vi "home arm.vi"(11 "Home":bool) -> ()   [LabVIEW 2017]
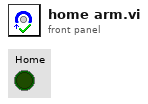
[diagram p1: front panel]
types:
  T1 = typedef "WPI_DigitalInputDevRef.ctl" = cluster{"DevStatus":errorcluster, "DIO Channel":T2}
  T2 = typedef "FPGA_DIOChannel.ctl" = enum8{"DIO 0", "DIO 1", "DIO 2", "DIO 3", "DIO 4", "DIO 5", "DIO 6", "DIO 7", "DIO 8", "DIO 9", "DIO MXP 0", "DIO MXP 1", "DIO MXP 2", "DIO MXP 3", "DIO MXP 4", "DIO MXP 5", "DIO MXP 6", "DIO MXP 7", "DIO MXP 8", "DIO MXP 9", "DIO MXP 10", "DIO MXP 11", "DIO MXP 12", "DIO MXP 13", "DIO MXP 14", "DIO MXP 15", "SPI Port CS1", "SPI Port CS2", "SPI Port CS3", "SPI Port MISO", "SPI Port MOSI", "Invalid"}
  T3 = typedef "WPI_MotorControlDeviceRef.ctl" = cluster{"DeviceStatus":errorcluster, "Type":T4, "PWM":cluster{"PWM Channel":T5, "DeadBand":T6}, "CAN":cluster{"Device Number":u8, "SetOutput VI Ref":variant, "GetOutput VI Ref":variant, "Enable VI Ref":variant, "Disable VI Ref":variant, "Data":variant}, "Invert":bool, "DIO PWM":cluster{"PWM \"Enable\" Channel":T5, "DIOChannel":T2, "PWM Rate":dbl}}
  T4 = typedef "WPI_MotorControlType.ctl" = enum16{"PWM", "CAN", "DIO PWM"}
  T5 = typedef "FPGA_DIOPWMChannel.ctl" = enum8{"PWM 0", "PWM 1", "PWM 2", "PWM 3", "PWM 4", "PWM 5", "PWM 6", "PWM 7", "PWM 8", "PWM 9", "PWM MXP 0", "PWM MXP 1", "PWM MXP 2", "PWM MXP 3", "PWM MXP 4", "PWM MXP 5", "PWM MXP 6", "PWM MXP 7", "PWM MXP 8", "PWM MXP 9", "Invalid"}
  T6 = typedef "WPI_PWMDeadband.ctl" = cluster{"Name":string, "maxPositivePwm":i32, "minPositivePwm":i32, "centerPwm":i32, "maxNegativePwm":i32, "minNegativePwm":i32, "angularRange":u16}
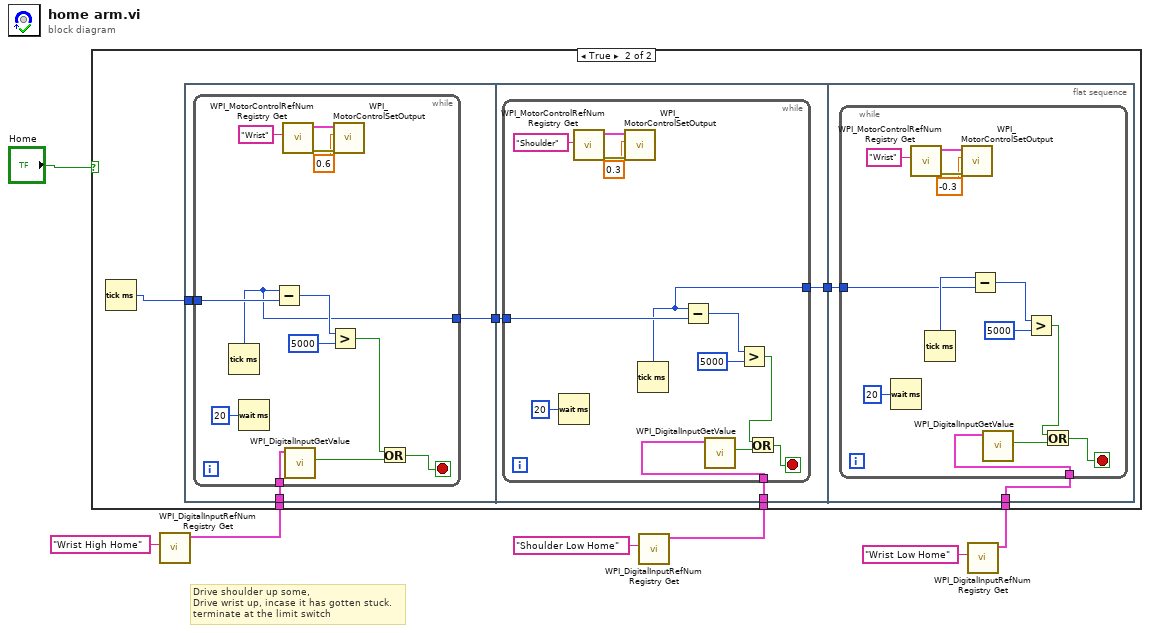
[diagram p0: block diagram]
diagram:
  # "Drive shoulder up some,\nDrive wrist up, incase it has gotten stuck.\nterminate at the limit switch"
  n1 = call <vilib>:"WPI_DigitalInputRefNum Registry Get.vi"("refnum name"="Wrist High Home") -> ("DigitalInputDevRef"=w6:T1)  [unwired: 9 in, 1 out]
  n2 = call <vilib>:"WPI_DigitalInputRefNum Registry Get.vi"("refnum name"="Shoulder Low Home") -> ("DigitalInputDevRef"=w3:T1)  [unwired: 9 in, 1 out]
  n3 = call <vilib>:"WPI_DigitalInputRefNum Registry Get.vi"("refnum name"="Wrist Low Home") -> ("DigitalInputDevRef"=w1:T1)  [unwired: 9 in, 1 out]
  n4 = case shown="True" "Home" {
    tunnel: w6 -> [_ w13]
    tunnel: w3 -> [_ w12]
    tunnel: w1 -> [_ w11]
    frame False {
    }
    frame True {
      n5 = Tick Count (ms)() -> (millisecond timer value=w10:u32)
      n6 = flat-sequence {
        tunnel: w13 -> [w16]
        tunnel: w10 -> [w15]
        tunnel: [w14] -> w9
        tunnel: w12 -> [w32]
        tunnel: w9 -> [w31]
        tunnel: [w30] -> w8
        tunnel: w11 -> [w47]
        tunnel: w8 -> [w46]
        frame #0 {
          n7 = while {
            tunnel: w16 -> [w23]
            tunnel: w15 -> [w21]
            tunnel: [w17] -> w14
            stop <- w25 stop-if-true
            n8 = Tick Count (ms)() -> (millisecond timer value=w17:u32)
            n9 = Wait (ms)(milliseconds to wait=u32 20) -> ()  [unwired: 1 out]
            n10 = Subtract(x=w17, y=w21) -> (x-y=w20:u32)
            n11 = call <vilib>:"WPI_MotorControlRefNum Registry Get.vi"("refnum name"="Wrist") -> ("error out"=w28:errorcluster, "MotorControlDevRef"=w27:T3)  [unwired: 9 in]
            n12 = call <vilib>:"WPI_DigitalInputGetValue.vi"("DigitalInputDevRef"=w23) -> ("Value"=w24:bool)  [unwired: 8 in, 2 out]
            n13 = Greater?(x=w20, y=u32 5000) -> (0:w18:bool)
            n14 = call <vilib>:"WPI_MotorControlSetOutput.vi"("error in (no error)"=w28, "Output"=0.6, "MotorControlDevRef"=w27) -> ()  [unwired: 6 in, 3 out]
            n15 = Or(x=w18, y=w24) -> (x .or. y?=w25:bool)
          }
        }
        frame #1 {
          n16 = while {
            tunnel: w32 -> [w41]
            tunnel: w31 -> [w35]
            tunnel: [w33] -> w30
            stop <- w39 stop-if-true
            n17 = Wait (ms)(milliseconds to wait=u32 20) -> ()  [unwired: 1 out]
            n18 = call <vilib>:"WPI_MotorControlRefNum Registry Get.vi"("refnum name"="Shoulder") -> ("error out"=w45:errorcluster, "MotorControlDevRef"=w44:T3)  [unwired: 9 in]
            n19 = call <vilib>:"WPI_MotorControlSetOutput.vi"("error in (no error)"=w45, "Output"=0.3, "MotorControlDevRef"=w44) -> ()  [unwired: 6 in, 3 out]
            n20 = Tick Count (ms)() -> (millisecond timer value=w33:u32)
            n21 = Subtract(x=w33, y=w35) -> (x-y=w37:u32)
            n22 = call <vilib>:"WPI_DigitalInputGetValue.vi"("DigitalInputDevRef"=w41) -> ("Value"=w40:bool)  [unwired: 8 in, 2 out]
            n23 = Greater?(x=w37, y=u32 5000) -> (0:w34:bool)
            n24 = Or(x=w34, y=w40) -> (x .or. y?=w39:bool)
          }
        }
        frame #2 {
          n25 = while {
            tunnel: w47 -> [w56]
            tunnel: w46 -> [w49]
            stop <- w54 stop-if-true
            n26 = Wait (ms)(milliseconds to wait=u32 20) -> ()  [unwired: 1 out]
            n27 = call <vilib>:"WPI_MotorControlRefNum Registry Get.vi"("refnum name"="Wrist") -> ("error out"=w59:errorcluster, "MotorControlDevRef"=w58:T3)  [unwired: 9 in]
            n28 = Tick Count (ms)() -> (millisecond timer value=w52:u32)
            n29 = call <vilib>:"WPI_MotorControlSetOutput.vi"("error in (no error)"=w59, "Output"=-0.3, "MotorControlDevRef"=w58) -> ()  [unwired: 6 in, 3 out]
            n30 = Subtract(x=w52, y=w49) -> (x-y=w51:u32)
            n31 = call <vilib>:"WPI_DigitalInputGetValue.vi"("DigitalInputDevRef"=w56) -> ("Value"=w55:bool)  [unwired: 8 in, 2 out]
            n32 = Greater?(x=w51, y=u32 5000) -> (0:w48:bool)
            n33 = Or(x=w48, y=w55) -> (x .or. y?=w54:bool)
          }
        }
      }
    }
  }
